vi "GetParam.vi"(8 "error in (no error)":errorcluster caption="entrée d'erreur (pas d'erreur)", 11 "Roc_Curve.lvclass":refnum<class "Roc_Curve.lvclass">) -> (0 "error out":errorcluster caption="sortie d'erreur", 2 "roc_curve":T1={"pos_label"={"dtype_pos_label"="None", "pos_label"="None"}, "sample_weight"=[], "drop_intermediate"=TRUE, "Returns"="fpr"}, 3 "Roc_Curve.lvclass":refnum<class "Roc_Curve.lvclass">)   [LabVIEW 2020, in "Roc_Curve.lvclass"]
doc: "Get Parameters"
uses:
  Roc_Curve.lvclass
  Roc_Curve.lvclass/Roc_Curve.ctl
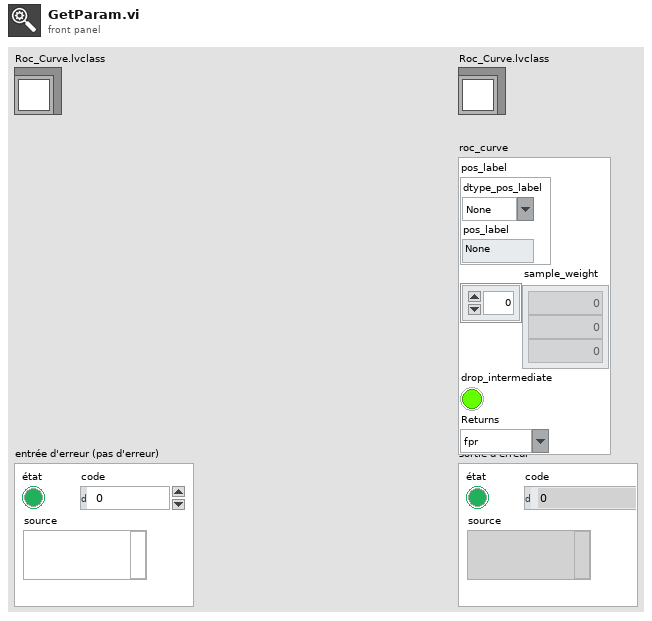
[diagram p1: front panel]
types:
  T1 = cluster{"pos_label":cluster{"dtype_pos_label":string, "pos_label":string}, "sample_weight":dbl[], "drop_intermediate":bool, "Returns":string}
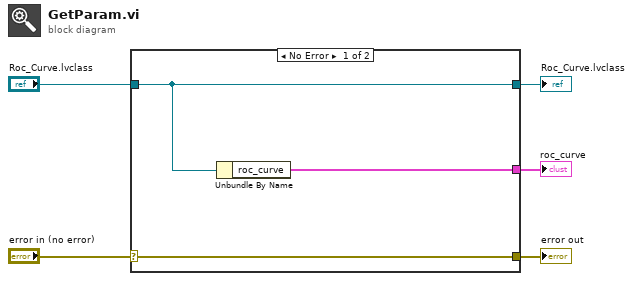
[diagram p0: block diagram]
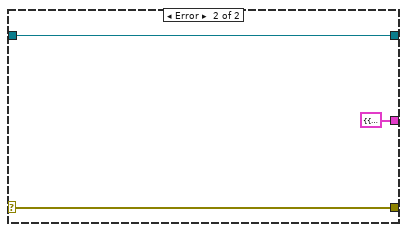
[diagram p2: hidden frame]
diagram:
  n1 = case shown="No Error" "error in (no error)" {
    selector: "error in (no error)" -> [w8 w10]
    tunnel: [w8 w10] -> w4
    tunnel: [w7 w11] -> w2
    tunnel: "Roc_Curve.lvclass" -> [w7 w11]
    tunnel: [w6 T1 {"pos_label"={"dtype_pos_label"="", "pos_label"=""}, "sample_weight"=[], "drop_intermediate"=FALSE, "Returns"=""} ("roc_curve")] -> w1
    frame No Error {
      n2 = Unbundle By Name(w7) -> ("roc_curve"=w6:T1)
    }
    frame Error {
    }
  }
  "error out" <- w4
  "Roc_Curve.lvclass" <- w2
  "roc_curve" <- w1
